vi "Register Logger.vi"(8 "error in (no error)":errorcluster, 9 "Task ID":string, 10 "EnQr":refnum<class "Message Enqueuer.lvclass">, 11 "LoggingManager in":refnum<class "LoggingManager.lvclass">) -> (0 "error out":errorcluster, 3 "LoggingManager out":refnum<class "LoggingManager.lvclass">)   [LabVIEW 2020, in "VolatusData.lvlib" / "LoggingManager.lvclass"]
uses:
  LoggingManager.lvclass
  LoggingManager.lvclass/LoggingManager.ctl
  Volatus/Task/Task.lvclass
  LoggingHandler Messages/Set Logging Root Msg/Set Logging Root Msg.lvclass
  C:/dev/lv20CE/relink/lv-volatus/Volatus/Task/Task.lvclass
  C:/Program Files (x86)/National Instruments/LabVIEW 2020/vi.lib/ActorFramework/Actor/Actor.lvclass
  C:/dev/lv20CE/relink/lv-volatus/Volatus/TaskStateHandler/TaskStateHandler.lvclass
  C:/dev/lv20CE/relink/lv-volatus/Volatus/VectoMessageHandler/VectoMessageHandler.lvclass
  C:/dev/lv20CE/relink/lv-volatus/VolatusData/LoggingManager/LoggingManager.lvclass
  C:/dev/lv20CE/relink/lv-volatus/Volatus/API Provider/API Provider.lvclass
  C:/dev/lv20CE/relink/lv-volatus/Volatus/RemoteCommandable/RemoteCommandable.lvclass
  C:/dev/lv20CE/relink/lv-volatus/VolatusData/LoggingHandler/LoggingHandler.lvclass
  <vilib>/ActorFramework/Message Enqueuer/Message Enqueuer.lvclass
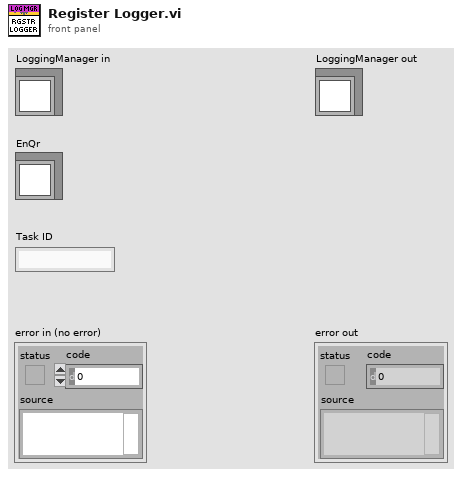
[diagram p1: front panel]
types:
  T1 = map{string, refnum<class "Message Enqueuer.lvclass">}
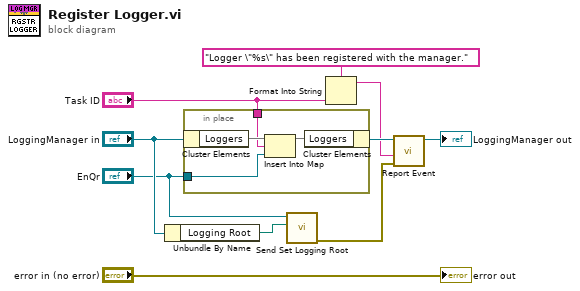
[diagram p0: block diagram]
diagram:
  n1 = Unbundle By Name("LoggingManager in") -> ("Logging Root"=w3:path)
  n2 = in-place {
    in-place-border: "Task ID" -> [w13]
    in-place-border: "EnQr" -> [w12]
    n3 = in-place-cluster #1("LoggingManager in") -> ("Loggers"=w14:T1)
    n4 = Insert Into Map(map in=w14, key=w13, value=w12) -> (map out=w11:T1)  [unwired: 2 out]
    n5 = in-place-cluster #1("Loggers"=w11) -> (w9:refnum<class "LoggingManager.lvclass">)
  }
  n6 = call "Send Set Logging Root.vi"("LoggingRoot"=w3, "Message Enqueuer"="EnQr") -> ("error out"=w1:errorcluster)  [unwired: 8 in, 1 out]
  n7 = Format Into String(format string="Logger \"%s\" has been registered with the manager.", "Task ID") -> (resulting string=w5:string)  [unwired: 2 in, 1 out]
  n8 = call "Report Event.vi"("error in (no error)"=w1, "Message"=w5, "Task in"=w9) -> ("Task out"=→"LoggingManager out":refnum<class "LoggingManager.lvclass">)  [unwired: 7 in, 1 out]
  "error out" <- "error in (no error)"
